vi "Destructor.vi"(8 "error in":errorcluster, 11 "OperationCycle in":refnum<class "OperationCycle.lvclass">) -> (0 "error out":errorcluster)   [LabVIEW 2021, in "ProligentXMLGenerator.lvlib" / "OperationCycle.lvclass"]
uses:
  OperationCycle.lvclass
  OperationCycle.lvclass/OperationCycle.ctl
  Model/CustomData/CustomData.lvclass
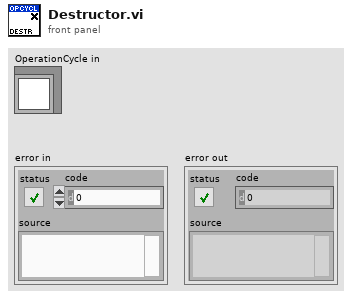
[diagram p1: front panel]
types:
  T1 = typedef "ProligentXMLGenerator.lvlib/OperationCycle.lvclass/Data.ctl" = cluster{"Name":string, "CustomData":refnum<class "CustomData.lvclass">, "ProcessFullName":refnum<class "ProcessFullName.lvclass">, "ProcessVersion":refnum<class "NonEmptyString_64.lvclass">, "OperationCycleId":refnum<class "Guid.lvclass">, "OperationName":refnum<class "NonEmptyString_65.lvclass">, "Location":refnum<class "FullName.lvclass">, "User":refnum<class "NonEmptyString_255.lvclass">, "OperationCycleStatus":refnum<class "ExecutionStatus.lvclass">, "OperationCycleStartTime":refnum<class "DateTime.lvclass">, "OperationCycleEndTime":refnum<class "DateTime.lvclass">, "TimeZoneInfoId":string}
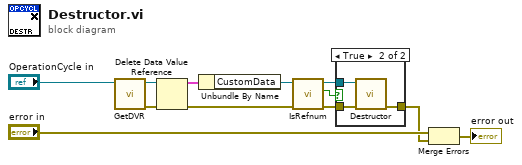
[diagram p0: block diagram]
diagram:
  n1 = call "GetDVR.vi"("OperationCycle in"="OperationCycle in") -> ("error out"=w9:errorcluster, "DVRReference"=w10:refnum<data-value>)  [unwired: 9 in]
  n2 = Delete Data Value Reference(data value reference=w10, error in=w9) -> (data value=w7:T1, error out=w1:errorcluster)
  n3 = Unbundle By Name(w7) -> ("CustomData"=w6:refnum<class "CustomData.lvclass">)
  n4 = call "IsRefnum.vi"("error in"=w1, "CustomDataType in"=w6) -> ("error out"=w3:errorcluster, "IsRefnum"=w5:bool, "CustomDataType out"=w4:refnum<class "CustomData.lvclass">)  [unwired: 7 in]
  n5 = case shown="True" w5 {
    tunnel: w4 -> [_ w16]
    tunnel: w3 -> [w13 w15]
    tunnel: [w13 w14] -> w2
    frame False {
    }
    frame True {
      n6 = call "Destructor.vi"("error in"=w15, "CustomDataType"=w16) -> ("error out"=w14:errorcluster)  [unwired: 9 in]
    }
  }
  n7 = Merge Errors("error in", w2) -> (→"error out":errorcluster)
